vi "Run Service.vi"(7 "measurement":refnum<class "Measurement Plugin Service.lvclass">, 8 "error in":errorcluster, 11 "measurementlink server user settings":T1={"stop server"=refnum, "measurement service versions"=[], "show front panel"=TRUE}) -> (0 "error out":errorcluster)   [LabVIEW 2021, in "NI Measurement Plug-In SDK.lvlib"]
uses:
  NI Measurement Plug-In SDK.lvlib
  Measurement Plugin Service/Measurement Plugin Service.lvclass
  Helpers/TypeDefs/Measurement Server User Settings.ctl
  Helpers/TypeDefs/Stop Server User Event.ctl
  Helpers/TypeDefs/Measurement Service Version.ctl
  <vilib>/gRPC/LabVIEW gRPC Servicer/Servicer/Servicer.lvclass/Servicer.ctl
  Clients/Discovery V1/Service Location FGV.vi
  IMeasurement Service/IMeasurement Service.lvclass
  <vilib>/gRPC/LabVIEW gRPC Servicer/Servicer/Servicer.lvclass
  gRPC/Generated APIs/ni/measurementlink/discovery/v1/ni.measurementlink.discovery.v1.api.lvlib
  Clients/Discovery V1/NI Discovery V1 Client.lvlib
panel:
  out "Display Name":string
  out "Listening Port":i32
  in  "Stop":bool
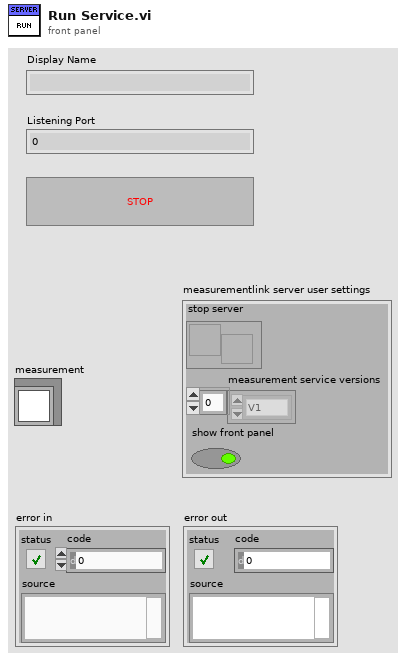
[diagram p1: front panel]
types:
  T1 = typedef "NI Measurement Plug-In SDK.lvlib/Measurement Server User Settings.ctl" = cluster{"stop server":T2, "measurement service versions":T3[], "show front panel":bool}
  T2 = typedef "NI Measurement Plug-In SDK.lvlib/Stop Server User Event.ctl" = refnum<user-event>
  T3 = typedef "NI Measurement Plug-In SDK.lvlib/Measurement Service Version.ctl" = enum16{"V1", "V2"}
  T4 = enum32{"Invalid", "Standard", "Closed", "Hidden", "Minimized", "Maximized"}
  T5 = typedef "NI Measurement Plug-In SDK.lvlib/Service Descriptor.ctl" = cluster{"measurement details":T6, "description URL":string, "service class":string, "measurement annotations":T7[]}
  T6 = typedef "NI Measurement Plug-In SDK.lvlib/Measurement Details.ctl" = cluster{"display name":string, "version":string}
  T7 = typedef "NI Measurement Plug-In SDK.lvlib/Measurement Annotation.ctl" = cluster{"key":string, "value":string}
  T8 = typedef "grpc-lvsupport-release.lvlib/grpcId.ctl" = u64
  T9 = typedef "ni.measurementlink.discovery.v1.api.lvlib/ni_measurementlink_discovery_v1_RegisterServiceResponse.ctl" = cluster{"registration_id":string}
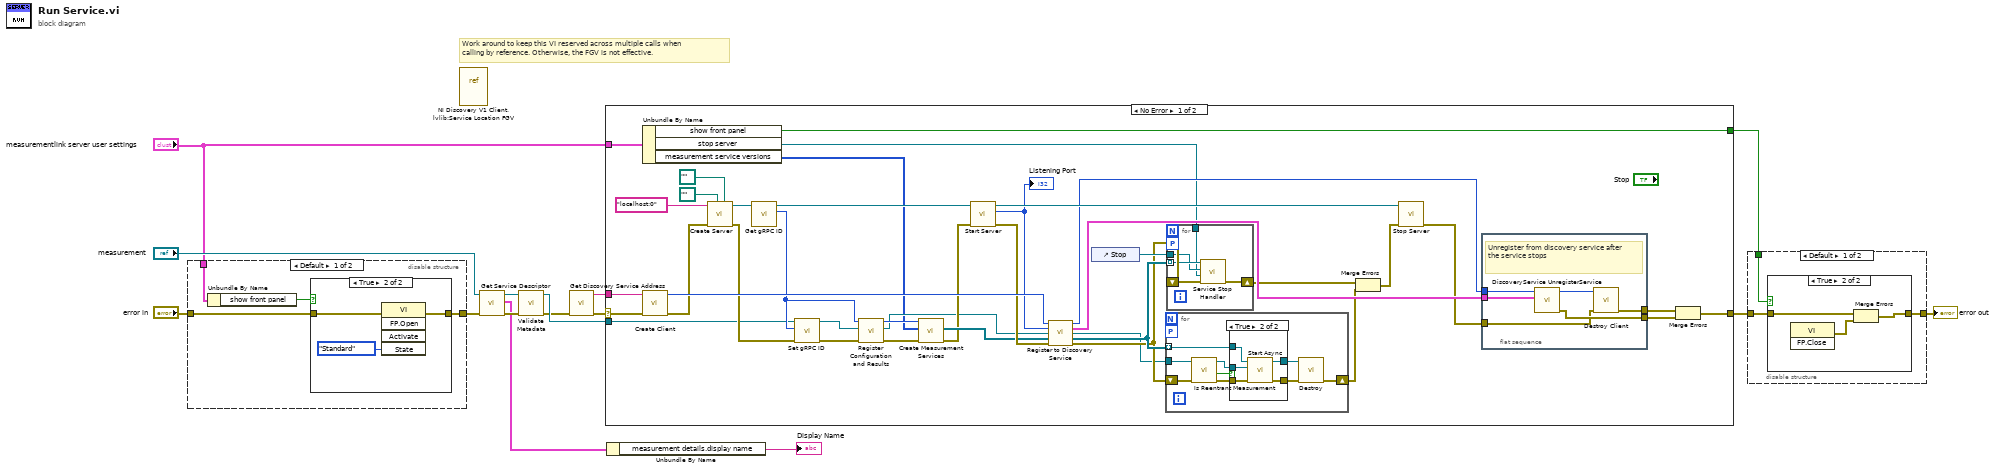
[diagram p0: block diagram]
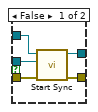
[diagram p6: hidden frame]
diagram:
  # "Work around to keep this VI reserved across multiple calls when\ncalling by reference. Otherwise, the FGV is not effective."
  n1 = disable-structure shown="Default" {
    disable-tunnel: [w19 w24] -> w12
    disable-tunnel: "error in" -> [w18 w24]
    disable-tunnel: "measurementlink server user settings" -> [w17 _]
    frame condition #0 (active) {
      n2 = Unbundle By Name(w17) -> ("show front panel"=w16:bool)
      n3 = case shown="True" w16 {
        tunnel: [w20 w22] -> w19
        tunnel: w18 -> [w20 w21]
        frame False {
          # "Don't show front panel when services are started using API."
        }
        frame True {
          n4 = invoke class="VI" method="FP.Open"(error in=w21, "State"=T4."Standard") -> (error out=w22:errorcluster)  [unwired: 3 in, 4 out]
        }
      }
    }
    frame condition #1 {
    }
  }
  n5 = vi-ref "NI Discovery V1 Client.lvlib:Service Location FGV.vi"() -> ()  [unwired: 1 out]
  n6 = call "Get Service Descriptor.vi"("error in"=w12, "measurement plugin service in"="measurement") -> ("error out"=w6:errorcluster, "service descriptor"=w4:T5, "measurement plugin service out"=w8:refnum<class "Measurement Plugin Service.lvclass">)  [unwired: 7 in]
  n7 = call "Validate Metadata.vi"("error in"=w6, "measurement plugin service in"=w8) -> ("error out"=w5:errorcluster, "measurement plugin service out"=w7:refnum<class "Measurement Plugin Service.lvclass">)  [unwired: 8 in]
  n8 = call "Get Discovery Service Address.vi"("error in"=w5) -> ("error out"=w15:errorcluster, "address"=w14:string)  [unwired: 9 in]
  n9 = case shown="No Error" w15 {
    selector: w15 -> [w29 w94]
    tunnel: [w63 w94] -> w10
    tunnel: w7 -> [w28 _]
    tunnel: w14 -> [w62 _]
    tunnel: "measurementlink server user settings" -> [w27 _]
    tunnel: [w25 _] -> w1
    frame No Error {
      n10 = Unbundle By Name(w27) -> ("show front panel"=w25:bool, "stop server"=w30:T2, "measurement service versions"=w26:T3[])
      n11 = call "Create Client.vi"("error in"=w29, "address"=w62) -> ("error out"=w51:errorcluster, "gRPC ID Out"=w55:T8)  [unwired: 8 in]
      n12 = call <vilib>:"Create Server.vi"("Server Key File (.key)"=path "", "Server Certificate File (.crt)"=path "", "error in"=w51, "Server Address"="localhost:0") -> ("error out"=w40:errorcluster, "gRPC server out"=w57:refnum<class "Servicer.lvclass">)  [unwired: 6 in]
      n13 = call <vilib>:"Get gRPC ID.vi"("gRPC server in"=w57) -> ("gRPC ID"=w38:T8, "gRPC server out"=w56:refnum<class "Servicer.lvclass">)  [unwired: 9 in]
      n14 = call "Set gRPC ID.vi"("error in"=w40, "gRPC ID"=w38, "measurement plugin service in"=w28) -> ("error out"=w39:errorcluster, "measurement plugin service out"=w37:refnum<class "Measurement Plugin Service.lvclass">)  [unwired: 7 in]
      n15 = call "Register Configuration and Results.vi"("error in"=w39, "measurement plugin service in"=w37, "gRPC ID in"=w38) -> ("error out"=w36:errorcluster, "measurement plugin service out"=w32:refnum<class "Measurement Plugin Service.lvclass">, "gRPC ID out"=w35:T8)  [unwired: 6 in]
      n16 = call "Create Measurement Services.vi"("error in"=w36, "measurement service versions"=w26, "gRPC ID in"=w35) -> ("error out"=w33:errorcluster, "measurement service array out"=w34:refnum<class "IMeasurement Service.lvclass">[])  [unwired: 6 in, 1 out]
      n17 = call <vilib>:"Start Server.vi"("error in"=w33, "gRPC server in"=w56) -> ("error out"=w48:errorcluster, "Listening Port"=w52:i32, "gRPC server out"=w61:refnum<class "Servicer.lvclass">)  [unwired: 7 in]
      "Listening Port" <- w52
      n18 = call "Register to Discovery Service.vi"("gRPC ID in"=w55, "port number"=w52, "measurement plugin service in"=w32, "measurement service in"=w34, "error in"=w48) -> ("gRPC ID out"=w54:T8, "response data"=w53:T9, "measurement plugin service out"=w31:refnum<class "Measurement Plugin Service.lvclass">, "measurement service out"=w44:refnum<class "IMeasurement Service.lvclass">[], "error out"=w43:errorcluster)  [unwired: 6 in]
      n19 = control-ref of="Stop"() -> (w45:refnum<vi>)
      n20 = for {
        workers-P: _ -> [_]
        tunnel: w44 -> [w72] mode=indexing
        tunnel: w31 -> [w65]
        shift-right: [w70] -> w42
        shift-left: w43 -> [w68]
        n21 = call "Is Reentrant Measurement.vi"("error in (no error)"=w68, "measurement plugin service in"=w65) -> ("error out"=w67:errorcluster, "is reentrant"=w66:bool, "measurement plugin service out"=w64:refnum<class "Measurement Plugin Service.lvclass">)  [unwired: 7 in]
        n22 = case shown="True" w66 {
          tunnel: w72 -> [w77 w79]
          tunnel: w64 -> [w76 w80]
          tunnel: [w75 w82] -> w71
          tunnel: [w74 w78] -> w69
          tunnel: w67 -> [w73 w81]
          frame False {
            n23 = call-dynamic "Start Sync.vi"("error in"=w73, "measurement plugin service in"=w76, "measurement service in"=w77) -> ("error out"=w75:errorcluster, "measurement service out"=w74:refnum<class "IMeasurement Service.lvclass">)  [unwired: 7 in]
          }
          frame True {
            n24 = call-dynamic "Start Async.vi"("error in (no error)"=w81, "measurement plugin service in"=w80, "measurement service in"=w79) -> ("error out"=w82:errorcluster, "measurement service out"=w78:refnum<class "IMeasurement Service.lvclass">)  [unwired: 7 in]
          }
        }
        n25 = call-dynamic "Destroy.vi"("error in"=w71, "measurement service in"=w69) -> ("error out"=w70:errorcluster)  [unwired: 9 in]
      }
      n26 = for {
        workers-P: _ -> [_]
        tunnel: w44 -> [w87] mode=indexing
        tunnel: w45 -> [w86]
        shift-right: [w84] -> w41
        shift-left: w43 -> [w85]
        tunnel: w30 -> [w83]
        n27 = call-dynamic "Service Stop Handler.vi"("error in"=w85, "stop server user event"=w83, "stop button ref"=w86, "measurement service in"=w87) -> ("error out"=w84:errorcluster)  [unwired: 6 in, 1 out]
      }
      n28 = Merge Errors(w41, w42) -> (w50:errorcluster)
      n29 = call <vilib>:"Stop Server.vi"("error in"=w50, "gRPC server in"=w61) -> ("error out"=w49:errorcluster)  [unwired: 9 in]
      n30 = flat-sequence {
        tunnel: w54 -> [w93]
        tunnel: w53 -> [w92]
        tunnel: [w91] -> w47
        tunnel: w49 -> [w88]
        tunnel: [w89] -> w46
        frame #0 {
          # "Unregister from discovery service after the service stops"
          n31 = call "DiscoveryService UnregisterService.vi"("Request Data"=w92, "gRPC ID"=w93) -> ("error out"=w89:errorcluster, "gRPC ID out"=w90:T8)  [unwired: 7 in, 1 out]
          n32 = call "Destroy Client.vi"("error in"=w88, "gRPC ID"=w90) -> ("error out"=w91:errorcluster)  [unwired: 9 in]
        }
      }
      n33 = Merge Errors(w47, w46) -> (w63:errorcluster)
    }
    frame Error {
    }
  }
  n34 = Unbundle By Name(w4) -> ("measurement details.display name"=→"Display Name":string)
  n35 = disable-structure shown="Default" {
    disable-tunnel: w10 -> [w97 w102]
    disable-tunnel: [w96 w102] -> w9
    disable-tunnel: w1 -> [w95 _]
    frame condition #0 (active) {
      n36 = case shown="True" w95 {
        tunnel: w97 -> [w98 w101]
        tunnel: [w98 w99] -> w96
        frame False {
        }
        frame True {
          n37 = invoke class="VI" method="FP.Close"() -> (error out=w100:errorcluster)  [unwired: 3 in, 2 out]
          n38 = Merge Errors(w101, w100) -> (w99:errorcluster)
        }
      }
    }
    frame condition #1 {
    }
  }
  "error out" <- w9
